vi "GEvt-Convert Filter Rules - v1.1.vi"(11 "Rules-v1":T1={"Global"={"CSM"=[], "LogType"=[], "State"=[], "StateType"=[]}, "CSM"={"LogType"=[], "State"=[], "StateType"=[]}, "PeriodicMessageFilter"={"Enable"=TRUE, "Threshold(#/s)"=2.0, "CheckPeriod(s)"=1.0}}) -> (3 "GlobalLogFilter":refnum<class "LogFilter.lvclass">)   [LabVIEW 2017, in "Communicable State Machine.lvlib"]
uses:
  Communicable State Machine.lvlib
  LogFilter/LogFilter.lvclass
  Typedef/_CSM_GlobalLog Filter Rules - v1.1.ctl
  Typedef/_CSM_GlobalLog_MSG_TYPE.ctl
  Typedef/_CSM_GlobalLog_STATE_TYPE.ctl
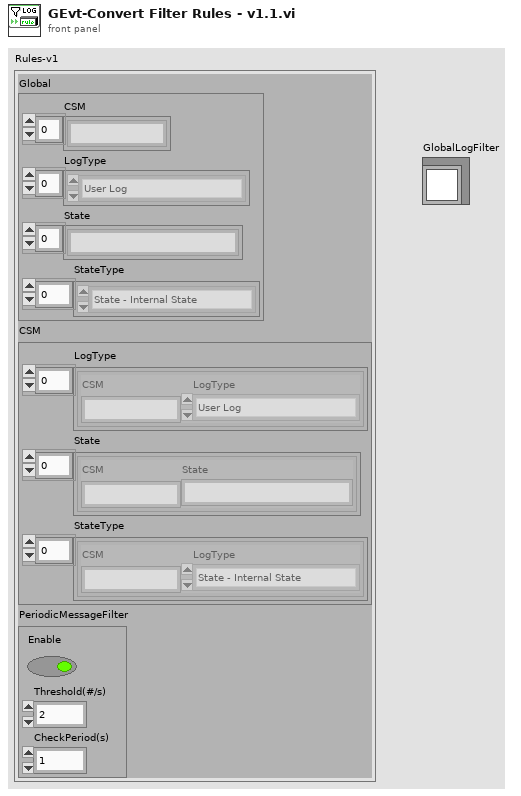
[diagram p1: front panel]
types:
  T1 = typedef "Communicable State Machine.lvlib/_CSM_GlobalLog Filter Rules - v1.1.ctl" = cluster{"Global":cluster{"CSM":string[], "LogType":T2[], "State":string[], "StateType":T3[]}, "CSM":cluster{"LogType":cluster{"CSM":string, "LogType":T2}[], "State":cluster{"CSM":string, "State":string}[], "StateType":cluster{"CSM":string, "LogType":T3}[]}, "PeriodicMessageFilter":cluster{"Enable":bool, "Threshold(#/s)":dbl, "CheckPeriod(s)":dbl}}
  T2 = typedef "Communicable State Machine.lvlib/_CSM_GlobalLog_MSG_TYPE.ctl" = enum16{"User Log", "State Change", "Status", "Interrupt", "Register", "Unregister", "Error Log", "Module Created", "Module Destroyed"}
  T3 = typedef "Communicable State Machine.lvlib/_CSM_GlobalLog_STATE_TYPE.ctl" = enum16{"State - Internal State", "State - External Message", "State - Response", "State - Complete"}
  T4 = cluster{"Enable":bool, "Threshold(#/s)":dbl, "CheckPeriod(s)":dbl}
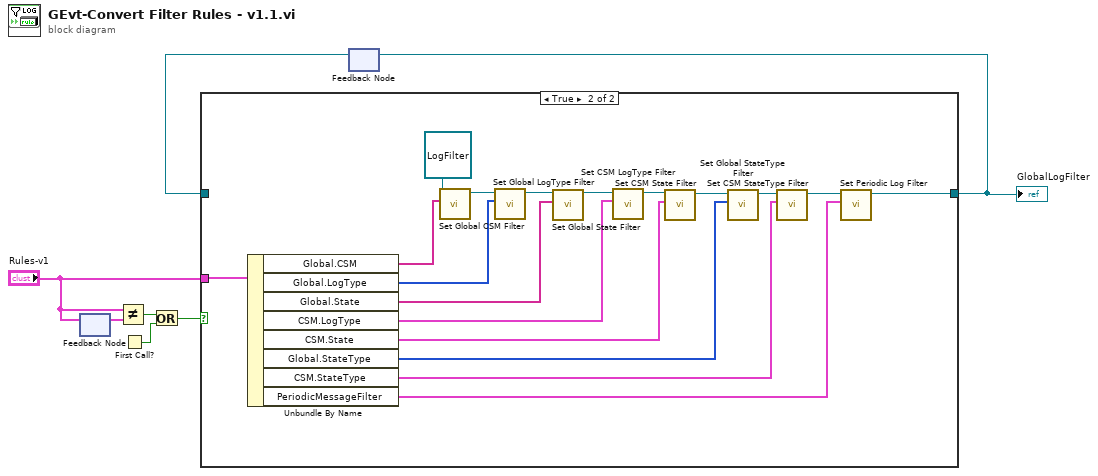
[diagram p0: block diagram]
diagram:
  n1 = feedback #1() -> (w2:T1)  [unwired: 1 in]
  n2 = feedback-in #1("Rules-v1") -> ()
  n3 = Not Equal?(x="Rules-v1", y=w2) -> (x != y?=w3:bool)
  n4 = First Call?() -> (First Call?: T/F=w4:bool)
  n5 = Or(x=w3, y=w4) -> (x .or. y?=w5:bool)
  n6 = feedback #2() -> (w7:refnum<class "LogFilter.lvclass">)  [unwired: 1 in]
  n7 = case shown="True" w5 {
    tunnel: [w8 w10] -> w6
    tunnel: "Rules-v1" -> [_ w22]
    tunnel: w7 -> [w8 _]
    frame False {
    }
    frame True {
      n8 = Unbundle By Name(w22) -> ("Global.CSM"=w24:string[], "Global.LogType"=w23:T2[], "Global.State"=w20:string[], "CSM.LogType"=w17:cluster{"CSM":string, "LogType":T2}[], "CSM.State"=w16:cluster{"CSM":string, "State":string}[], "Global.StateType"=w12:T3[], "CSM.StateType"=w11:cluster{"CSM":string, "LogType":T3}[], "PeriodicMessageFilter"=w9:T4)
      n9 = call "Set Global CSM Filter.vi"("Group:CSM"=w24, "GlobalLogFilter In"=refnum<class "LogFilter.lvclass"> refnum ("GlobalLogFilter.lvclass")) -> ("GlobalLogFilter Out"=w25:refnum<class "LogFilter.lvclass">)  [unwired: 9 in]
      n10 = call "Set Global LogType Filter.vi"("Group:LogType"=w23, "GlobalLogFilter In"=w25) -> ("GlobalLogFilter Out"=w21:refnum<class "LogFilter.lvclass">)  [unwired: 9 in]
      n11 = call "Set Global State Filter.vi"("Group:State"=w20, "GlobalLogFilter In"=w21) -> ("GlobalLogFilter Out"=w18:refnum<class "LogFilter.lvclass">)  [unwired: 9 in]
      n12 = call "Set CSM LogType Filter.vi"("LogType"=w17, "GlobalLogFilter In"=w18) -> ("GlobalLogFilter Out"=w19:refnum<class "LogFilter.lvclass">)  [unwired: 9 in]
      n13 = call "Set CSM State Filter.vi"("CSM:State"=w16, "GlobalLogFilter In"=w19) -> ("GlobalLogFilter Out"=w14:refnum<class "LogFilter.lvclass">)  [unwired: 9 in]
      n14 = call "Set Global StateType Filter.vi"("Group:LogType"=w12, "GlobalLogFilter In"=w14) -> ("GlobalLogFilter Out"=w15:refnum<class "LogFilter.lvclass">)  [unwired: 9 in]
      n15 = call "Set CSM StateType Filter.vi"("LogType"=w11, "GlobalLogFilter In"=w15) -> ("GlobalLogFilter Out"=w13:refnum<class "LogFilter.lvclass">)  [unwired: 9 in]
      n16 = call "Set Periodic Log Filter.vi"("PeriodicLogFilter"=w9, "GlobalLogFilter In"=w13) -> ("GlobalLogFilter Out"=w10:refnum<class "LogFilter.lvclass">)  [unwired: 9 in]
    }
  }
  "GlobalLogFilter" <- w6
  n17 = feedback-in #2(w6) -> ()
